vi "Get State.vi"(8 "error in (no error)":errorcluster) -> (0 "error out":errorcluster, 2 "Data":variant, 3 "Next State":T1=enum."SCAN")   [LabVIEW 2014]
uses:
  Controls/StateControl.ctl
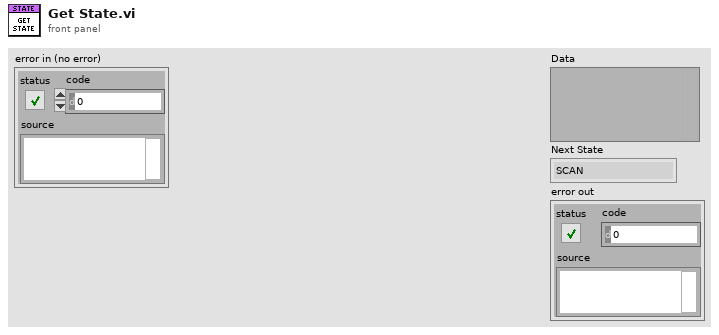
[diagram p1: front panel]
types:
  T1 = typedef "StateControl.ctl" = enum16{"WAIT FOR EVENT", "GET HEALTH", "SCAN", "RESET", "EXIT"}
  T2 = typedef "State Typedef.ctl" = cluster{"State":T1, "Data":variant}
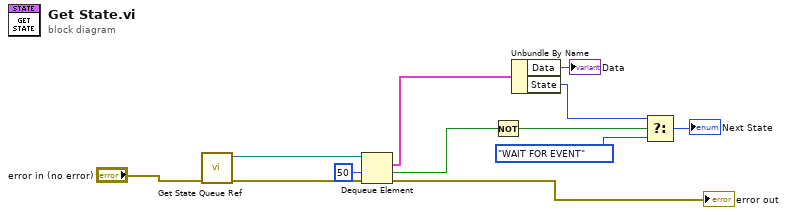
[diagram p0: block diagram]
diagram:
  n1 = call "Get State Queue Ref.vi"("error in (no error)"="error in (no error)") -> ("error out"=w11:errorcluster, "queue out"=w9:refnum<queue>)  [unwired: 9 in]
  n2 = Dequeue Element(queue=w9, timeout in ms (-1)=50, error in (no error)=w11) -> (element=w7:T2, timed out?=w8:bool, error out=→"error out":errorcluster)  [unwired: 1 out]
  n3 = Not(x=w8) -> (.not. x?=w6:bool)
  n4 = Unbundle By Name(w7) -> ("Data"=→"Data":variant, "State"=w5:T1)
  n5 = Select(t=w5, s=w6, f=StateControl."WAIT FOR EVENT") -> (s? t:f=→"Next State":T1)
